vi "iWorx - Heart Sounds.vi"() -> ()   [LabVIEW 2012]
uses:
  <vilib>/DAQmx/create/channels.llb/DAQmx Create Channel (AI-Voltage-Basic).vi
  <vilib>/DAQmx/read.llb/DAQmx Read (Analog 1D Wfm NChan 1Samp).vi
  <vilib>/DAQmx/configure/timing.llb/DAQmx Timing (Sample Clock).vi
  <vilib>/measure/NI_MAPro.lvlib
  <vilib>/measure/macond.llb/IIR Filter for 1 Chan.vi
  vi.lib/iWorx/iWorx Set Points.ctl
panel:
  out "error out":errorcluster
  in  "Reset Default Cal":bool
  in  "Set Points":T1={"SP1 Voltage"=0.0, "SP1 Value"=0.0, "SP2 Voltage"=1.0, "SP2 Value"=26.4} {"SP2 Value" format="%.1f mmH20"; "SP2 Voltage" format="%.2f V"; "SP1 Value" format="%.0f mmH20"; "SP1 Voltage" format="%.2f V"}
  out "Offset(b)":dbl
  out "Slope(m)":dbl=26.4
  in  "Reset Scale":bool
  in  "Stop":bool
  in  "Log Info Button":bool
  in  "Set Up":bool
  in  "Channel":u16(ring) items=["Channel 1", "Channel 2"]
  in  "Pause Button":bool
  in  "Snapshot":bool
  out "Processed Signal":dbl(knob) caption="Pressue" scale=-20.0..20.0
  out "Waveform Chart":waveform(dbl)(graph)
  in  "Clear Chart":bool
  in  "Open Log":bool
  in  "Rescale Y":bool
  out "Raw Signal":dbl(knob) scale=-10.0..10.0
  # "iWorx - Heart Sounds - Data Logger"
  # "Sensor Input"
  # "(            ,              )"
  # "(            ,              )"
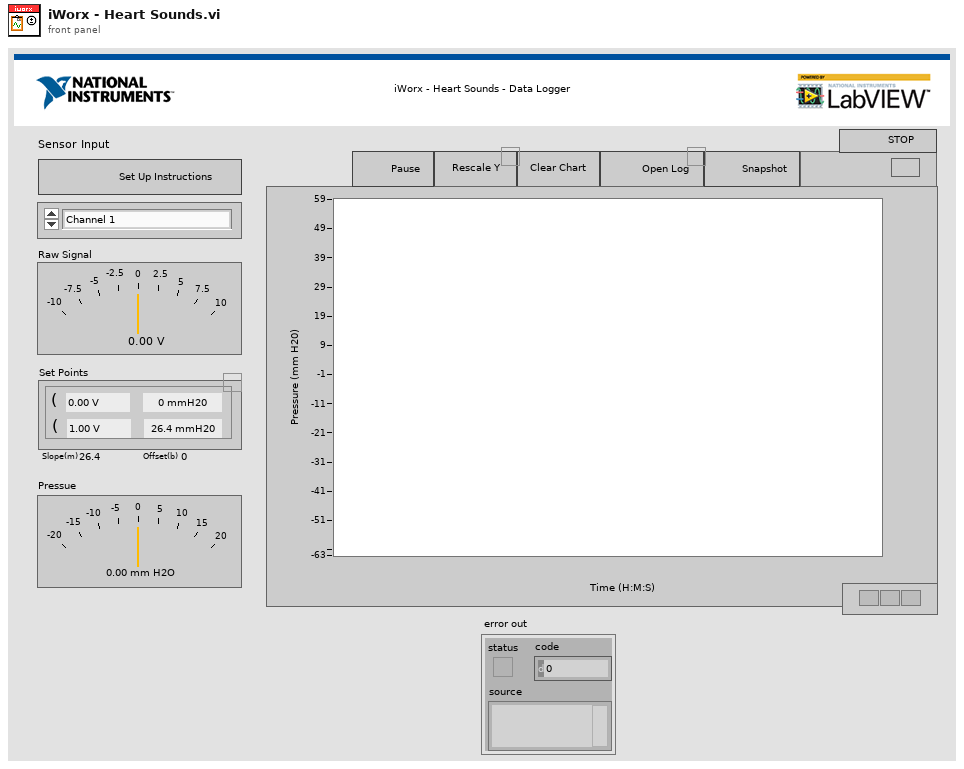
[diagram p1: front panel]
types:
  T1 = typedef "iWorx Set Points.ctl" = cluster{"SP1 Voltage":dbl, "SP1 Value":dbl, "SP2 Voltage":dbl, "SP2 Value":dbl}
  T2 = cluster{"Topology":enum16{"Off", "Butterworth", "Chebyshev", "Inverse Chebyshev", "Elliptic", "Bessel"}, "Type":enum16{"Lowpass", "Highpass", "Bandpass", "Bandstop"}, "Order":i32, "Lower Fc":dbl, "Upper Fc":dbl, "PB Ripple":dbl, "SB Attenuation":dbl}
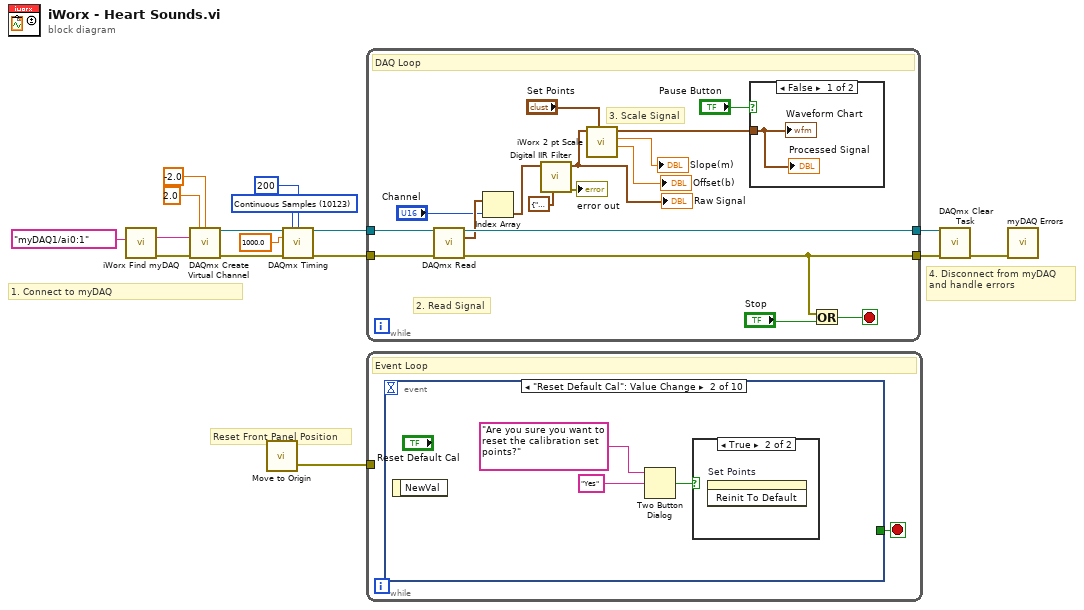
[diagram p0: block diagram]
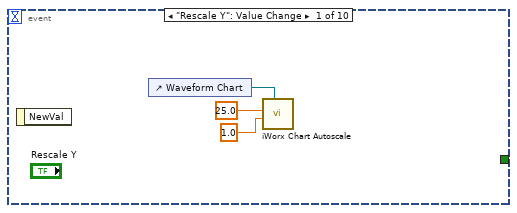
[diagram p2: hidden frame]
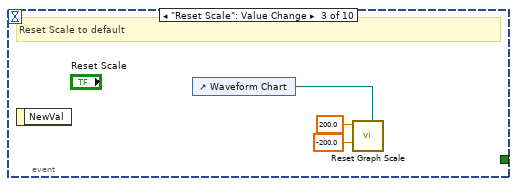
[diagram p4: hidden frame]
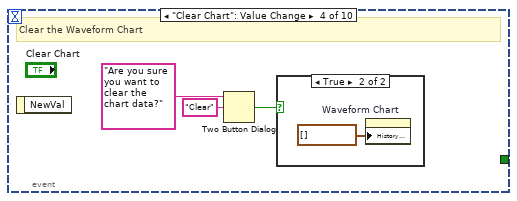
[diagram p5: hidden frame]
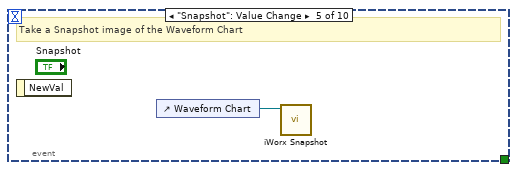
[diagram p7: hidden frame]
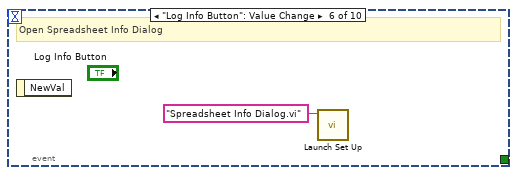
[diagram p8: hidden frame]
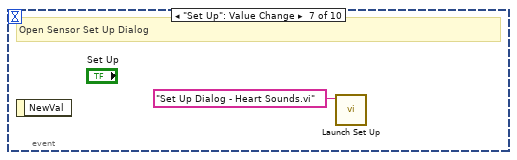
[diagram p9: hidden frame]
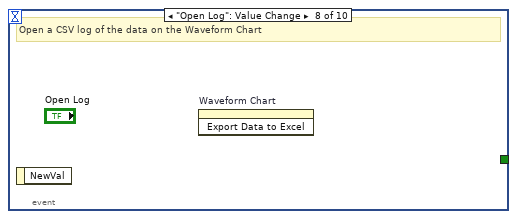
[diagram p10: hidden frame]
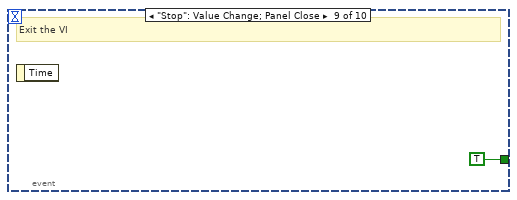
[diagram p11: hidden frame]
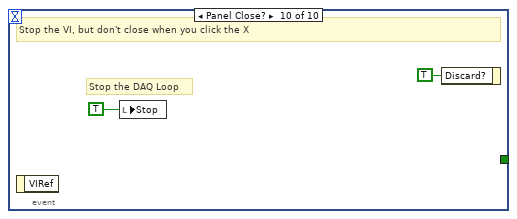
[diagram p12: hidden frame]
diagram:
  w7 = 10123 items=["Finite Samples"=10178, "Continuous Samples"=10123, "Hardware Timed Single Point"=12522] ("sample mode")
  # "Reset Front Panel Position"
  # "4. Disconnect from myDAQ and handle errors"
  # "1. Connect to myDAQ"
  n1 = call "iWorx Find myDAQ.vi"("Preferred myDAQ (myDAQ1)"=tag "myDAQ1/ai0:1") -> ("Error Out"=w12:errorcluster, "DAQmx Physical Channel"=w13:tag)  [unwired: 6 in, 3 out]
  n2 = call-poly <vilib>:"DAQmx Create Virtual Channel.vi"("maximum value"=2.0, "minimum value"=-2.0, "physical channels"=w13, "error in"=w12) -> ("task out"=w5:refnum<k21>, "error out"=w2:errorcluster)  [unwired: 10 in]
  n3 = call "Move to Origin.vi"() -> ("Error Out"=w10:errorcluster)  [unwired: 3 in]
  n4 = call-poly <vilib>:"DAQmx Timing.vi"("task/channels in"=w5, "sample mode"=w7, "samples per channel"=200, "rate"=1000.0, "error in"=w2) -> ("task out"=w4:refnum<k21>, "error out"=w3:errorcluster)  [unwired: 9 in]
  n5 = while {
    tunnel: w4 -> [w33]
    tunnel: [w32] -> w16
    tunnel: w3 -> [w31]
    tunnel: [w29] -> w15
    stop <- w30 stop-if-true
    # "3. Scale Signal"
    # "2. Read Signal"
    # "DAQ Loop"
    n6 = call-poly <vilib>:"DAQmx Read.vi"("task/channels in"=w33, "error in"=w31) -> ("task out"=w32:refnum<k21>, "data"=w27:waveform(dbl)[], "error out"=w29:errorcluster)  [unwired: 11 in]
    n7 = Index Array(array=w27, index="Channel") -> (element=w18:waveform(dbl))
    n8 = call-poly <vilib>:"Digital IIR Filter.vi"("IIR filter specifications"=T2 {"Topology"=enum."Butterworth", "Type"=enum."Lowpass", "Order"=2, "Lower Fc"=20.0, "Upper Fc"=200.0, "PB Ripple"=1.0, "SB Attenuation"=60.0}, "signal in"=w18) -> ("error out"=→"error out":errorcluster, "signal out"=w17:waveform(dbl))  [unwired: 7 in, 1 out]
    "Raw Signal" <- w17
    n9 = call "iWorx 2 pt Scale.vi"("Set Points"="Set Points", "Raw Waveform"=w17) -> ("Offset"=→"Offset(b)":dbl, "Slope"=→"Slope(m)":dbl, "Scaled Value"=w26:waveform(dbl))  [unwired: 7 in]
    n10 = case shown="False" "Pause Button" {
      tunnel: w26 -> [w34 _]
      frame False {
        "Waveform Chart" <- w34
        "Processed Signal" <- w34
      }
      frame True {
        # "Do Not update controls"
      }
    }
    n11 = Or(x=w29, y="Stop") -> (x .or. y?=w30:bool)
  }
  n12 = while {
    tunnel: w10 -> [_]
    stop <- w35 stop-if-true
    # "Event Loop"
    n13 = event shown="[1] \"Reset Default Cal\": Value Change" {
      selector: _ -> [_ _ _ _ _ _ _ _ _ _]
      dyn-events: _ -> [_ _ _ _ _ _ _ _ _ _]
      timeout: _ -> [_ _ _ _ _ _ _ _ _ _]
      tunnel: [_ _ _ _ _ _ _ _ TRUE _] -> w35
      event "Rescale Y": Value Change {
        n14 = event-data() -> ()  [unwired: 1 in, 1 out]
        n15 = control-ref of="Waveform Chart"() -> (w38:refnum<vi>)
        n16 = call "iWorx Chart Autoscale.vi"("Selection Chart"=w38, "Rounding Multiple (10)"=1.0 ("Rounding Multiple (1)"), "Padding (10%)"=25.0 ("Rounding Multiple (1)")) -> ()  [unwired: 6 in, 3 out]
      }
      event "Reset Default Cal": Value Change {
        n17 = event-data() -> ()  [unwired: 1 in, 1 out]
        n18 = Two Button Dialog(message="Are you sure you want to reset the calibration set points?", 2:"Yes" ("T button name (\"OK\")")) -> (T button?=w39:bool)  [unwired: 1 in]
        n19 = case shown="True" w39 {
          frame False {
          }
          frame True {
            n20 = invoke on="Set Points" class="Clust (strict)" method="Reinit To Default"() -> ()  [unwired: 3 in, 3 out]
          }
        }
      }
      event "Reset Scale": Value Change {
        # "Reset Scale to default"
        n21 = event-data() -> ()  [unwired: 1 in, 1 out]
        n22 = control-ref of="Waveform Chart"() -> (w44:refnum<vi>)
        n23 = call "Reset Graph Scale.vi"("WaveformChart in"=w44, "Minimum (0)"=-200.0, "Maximum (100)"=200.0) -> ()  [unwired: 8 in, 1 out]
      }
      event "Clear Chart": Value Change {
        # "Clear the Waveform Chart"
        n24 = event-data() -> ()  [unwired: 1 in, 1 out]
        n25 = Two Button Dialog(message="Are you sure you want to clear the chart data?", 2:"Clear" ("T button name (\"OK\")")) -> (T button?=w46:bool)  [unwired: 1 in]
        n26 = case shown="True" w46 {
          frame False {
          }
          frame True {
            n27 = property on="Waveform Chart" class="WFChart (strict)"("History Data"=waveform(dbl)[] []) -> ()  [unwired: 2 in, 2 out]
          }
        }
      }
      event "Snapshot": Value Change {
        # "Take a Snapshot image of the Waveform Chart"
        n28 = event-data() -> ()  [unwired: 1 in, 1 out]
        n29 = control-ref of="Waveform Chart"() -> (w49:refnum<vi>)
        n30 = call "iWorx Snapshot.vi"("WaveformChart in"=w49) -> ()  [unwired: 10 in, 1 out]
      }
      event "Log Info Button": Value Change {
        # "Open Spreadsheet Info Dialog"
        n31 = event-data() -> ()  [unwired: 1 in, 1 out]
        n32 = call "Launch Set Up.vi"("name or relative path"="Spreadsheet Info Dialog.vi") -> ()  [unwired: 9 in, 2 out]
      }
      event "Set Up": Value Change {
        # "Open Sensor Set Up Dialog"
        n33 = event-data() -> ()  [unwired: 1 in, 1 out]
        n34 = call "Launch Set Up.vi"("name or relative path"="Set Up Dialog - Heart Sounds.vi") -> ()  [unwired: 9 in, 2 out]
      }
      event "Open Log": Value Change {
        # "Open a CSV log of the data on the Waveform Chart"
        n35 = event-data() -> ()  [unwired: 1 in, 1 out]
        n36 = invoke on="Waveform Chart" class="WFChart (strict)" method="Export Data to Excel"() -> ()  [unwired: 3 in, 3 out]
      }
      event "Stop": Value Change; Panel Close {
        # "Exit the VI"
        n37 = event-data() -> ()  [unwired: 1 in, 1 out]
      }
      event Panel Close? {
        # "Stop the DAQ Loop"
        # "Stop the VI, but don't close when you click the X"
        n38 = event-data() -> ()  [unwired: 1 in, 1 out]
        n39 = local write "Stop"(TRUE ("stop")) -> ()
        n40 = event-data("Discard?"=TRUE) -> ()  [unwired: 1 in, 1 out]
      }
    }
  }
  n41 = call <vilib>:"DAQmx Clear Task.vi"("task in"=w16, "error in"=w15) -> ("error out"=w14:errorcluster)  [unwired: 13 in]
  n42 = call "myDAQ Errors.vi"("error in (no error)"=w14) -> ()  [unwired: 10 in, 1 out]
